vi "Unpack Panel Close.vi"(11 "PanelCloseMsg in":refnum<class "PanelCloseMsg.lvclass">) -> (2 "Discarded?":bool, 3 "Name":string)   [LabVIEW 2015, in "ActorAutoRegistration.lvlib" / "PanelCloseMsg.lvclass"]
uses:
  PanelCloseMsg.lvclass
  PanelCloseMsg.lvclass/PanelCloseMsg.ctl
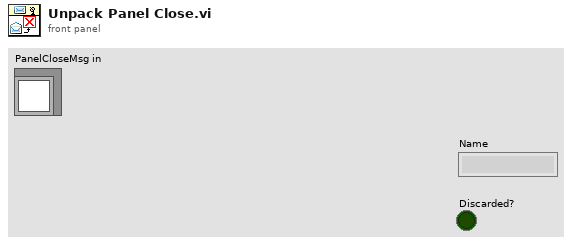
[diagram p1: front panel]
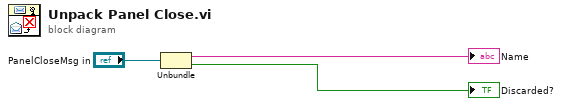
[diagram p0: block diagram]
diagram:
  n1 = Unbundle("PanelCloseMsg in") -> (→"Name":string, →"Discarded?":bool)
